vi "Create Enums For Registration.vi"(8 "error in (no error)":errorcluster, 10 "Enum MetaData":T1[](array[typedef]), 11 "VI in":refnum<vi>) -> (0 "error out":errorcluster, 3 "VI out":refnum<vi>)   [LabVIEW 2019, in "gRPC Template Creation Utility.lvlib"]
uses:
  gRPC Template Creation Utility.lvlib
  TypeDefs/Enum Metadata (Scripting).ctl
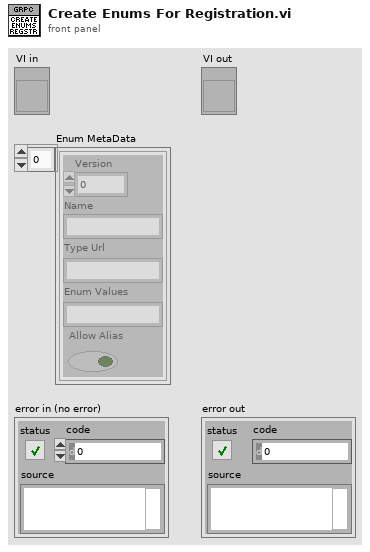
[diagram p1: front panel]
types:
  T1 = typedef "gRPC Template Creation Utility.lvlib/Enum Metadata (Scripting).ctl" = cluster{"Version":i32, "Name":string, "Type Url":string, "Enum Values":string, "Allow Alias":bool}
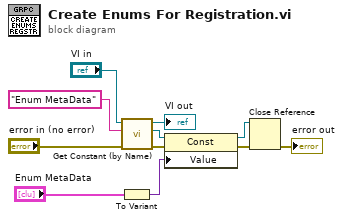
[diagram p0: block diagram]
diagram:
  n1 = call "Get Constant (by Name).vi"("error in (no error)"="error in (no error)", "Constant Label"="Enum MetaData", "Owner VI in"="VI in") -> ("error out"=w8:errorcluster, "Const ref out"=w9:refnum<vi>, "Owner VI out"=→"VI out":refnum<vi>)  [unwired: 5 in, 1 out]
  n2 = To Variant(anything="Enum MetaData") -> (Variant=w6:variant)
  n3 = property class="Const"(reference=w9, error in=w8, "Value"=w6) -> (reference out=w11:refnum<vi>, error out=w10:errorcluster)
  n4 = Close Reference(reference=w11, error in (no error)=w10) -> (error out=→"error out":errorcluster)
